vi "Unflatten UIP Value.vi"(10 "String Value":string, 11 "Disabled UIP In":refnum<class "DisabledUIP.lvclass">) -> (0 "Error Out":errorcluster, 3 "Disabled UIP Out":refnum<class "DisabledUIP.lvclass">)   [LabVIEW 2015, in "DisabledUIP.lvclass"]
uses:
  DisabledUIP.lvclass
  DisabledUIP.lvclass/DisabledUIP.ctl
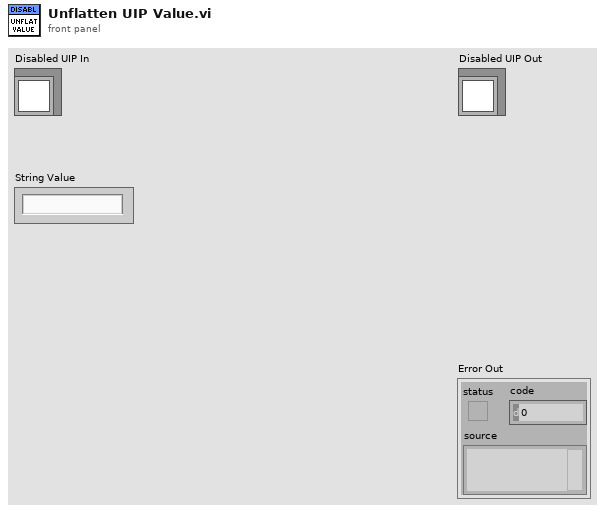
[diagram p1: front panel]
types:
  T1 = enum8{"Enabled", "Disabled", "Disabled and Grayed Out"}
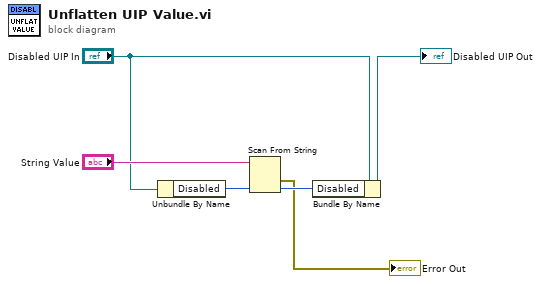
[diagram p0: block diagram]
diagram:
  n1 = Unbundle By Name("Disabled UIP In") -> ("Disabled"=w5:T1)
  n2 = Scan From String(input string="String Value", default 1=w5) -> (error out=→"Error Out":errorcluster, output 1=w2:T1)  [unwired: 3 in, 2 out]
  n3 = Bundle By Name(cluster="Disabled UIP In", "Disabled"=w2) -> (→"Disabled UIP Out":refnum<class "DisabledUIP.lvclass">)
